vi "Test Program.vi"() -> ()   [LabVIEW 2018]
uses:
  <vilib>/Analysis/Matrix/Datatypes/RealMatrix.ctl
  archive/CAEN_SY527 v3/CAEN_SY527/CAEN globals.vi
  <vilib>/Analysis/Matrix/NI_Matrix.lvlib
panel:
  in  "Mainframe 2":refnum<visa-resource-name>
  in  "Buffer":T1(ring)=enum."None"
  in  "Action":string(combo)
  in  "Read Port":bool
  in  "Predefined Range":T2(ring)
  in  "Combo funcs":bool
  in  "Write Voltage":bool
  in  "Current Limit (mA)":i32
  in  "Write Current Lim":bool
  in  "Read All":bool
  out "Channel+range":string
  in  "Voltage (V)":i32
  out "Codes Output":string
  in  "Connect to Crate":bool
  out "Channel Read as Matrix":T3
  out "Serial Readout":string
  in  "Abort and Clear":bool
  in  "stop":bool
  in  "Range Source":enum16{"Predefined Range", "Selected Range"}(ring)
  in  "Crate":i32=1
  in  "Card":i32
  in  "Channel":i32
  in  "# Channels":i32
  in  "Read Range":bool
  out "Errors":errorcluster
  in  "Mainframe 1":refnum<visa-resource-name>
  # "Select Channel Range to Operate On"
  # "Write Operations"
  # "Read Operations"
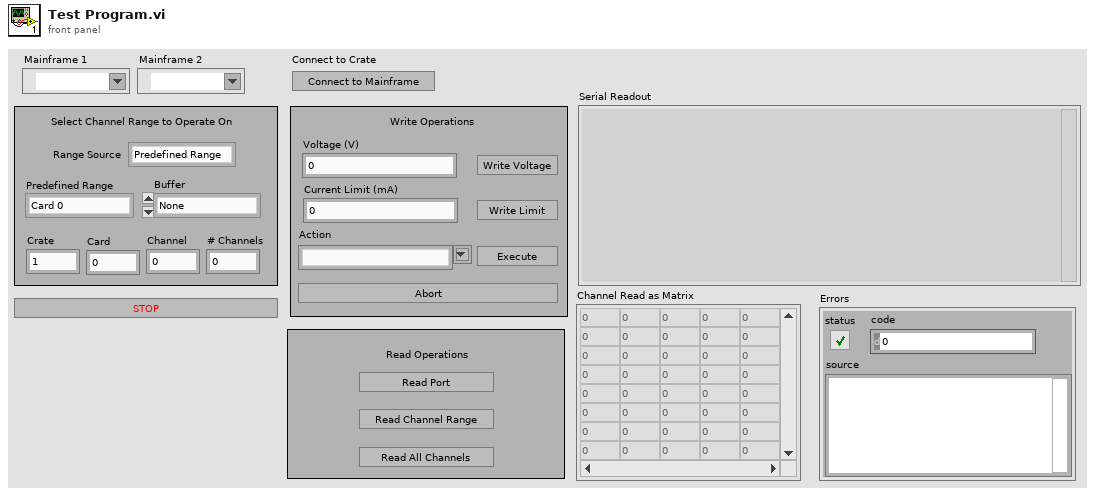
[diagram p1: front panel]
types:
  T1 = enum16{"Monitor", "Demand", "Backup", "All", "None"}
  T2 = enum16{"Card 0", "Card 1", "Card 2", "Card 3", "Card 4", "Card 5", "Card 6", "Card 7", "Card 8", "Card 9", "Card 10", "Card 11", "Card 12", "Card 13", "Card 14", "Card 15"}
  T3 = typedef "NI_Matrix.lvlib/RealMatrix.ctl" = dbl[][]
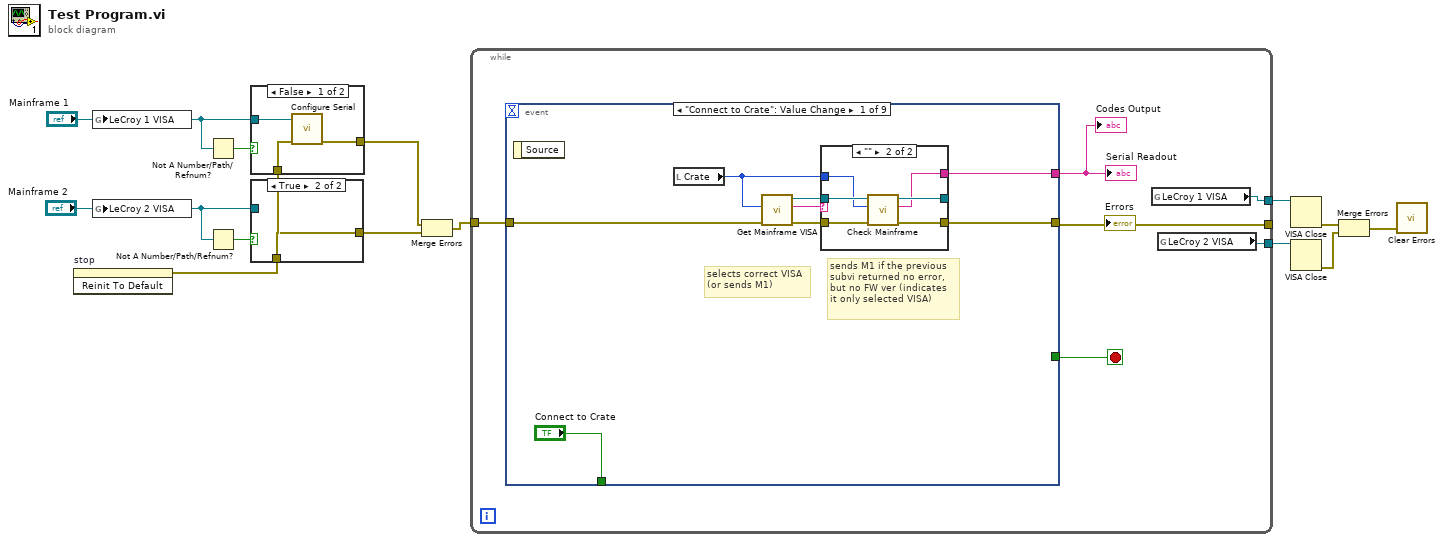
[diagram p0: block diagram]
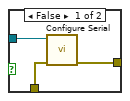
[diagram p2: hidden frame]
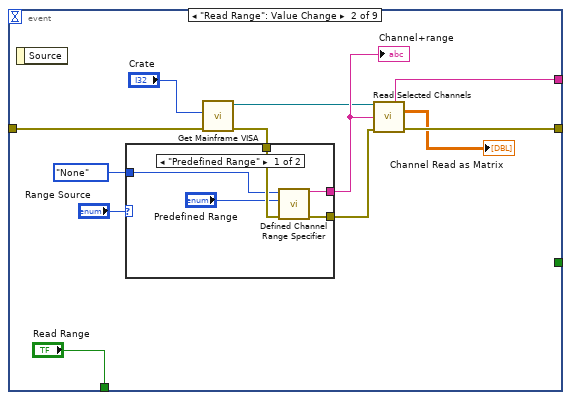
[diagram p5: hidden frame]
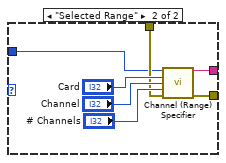
[diagram p6: hidden frame]
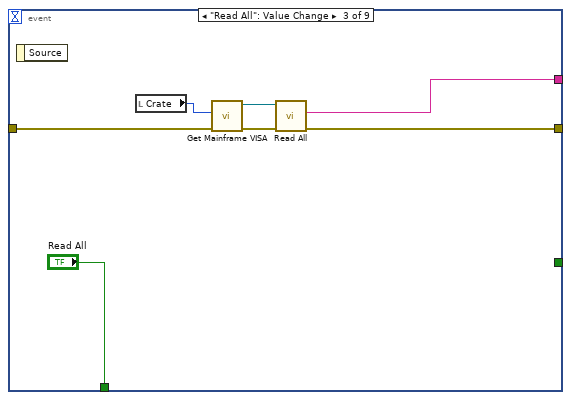
[diagram p7: hidden frame]
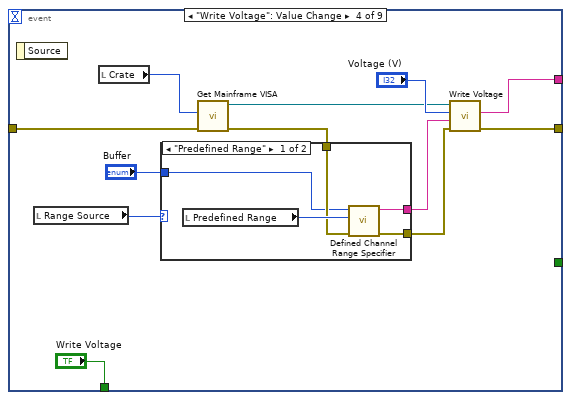
[diagram p8: hidden frame]
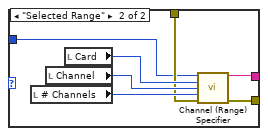
[diagram p9: hidden frame]
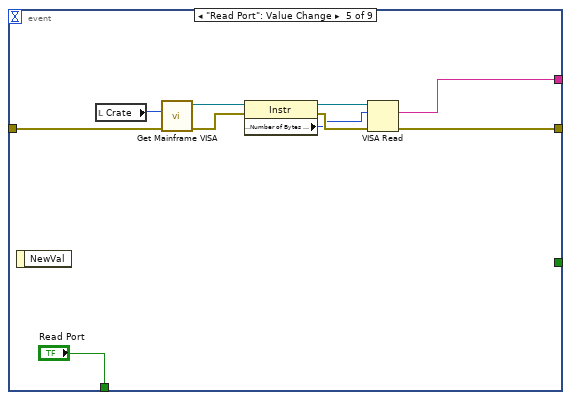
[diagram p10: hidden frame]
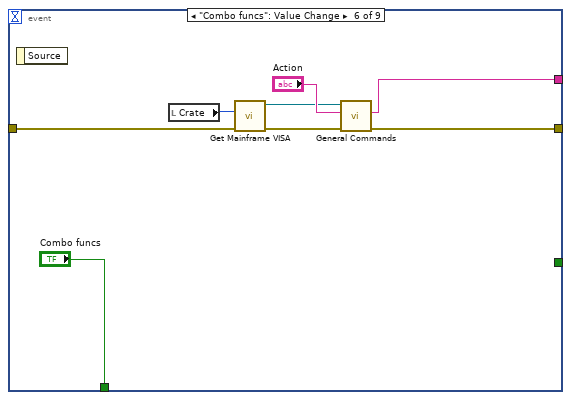
[diagram p11: hidden frame]
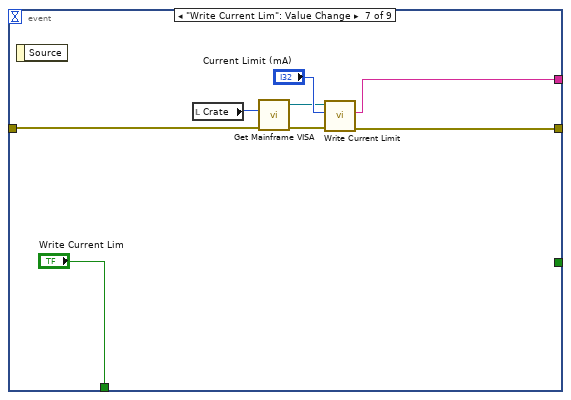
[diagram p12: hidden frame]
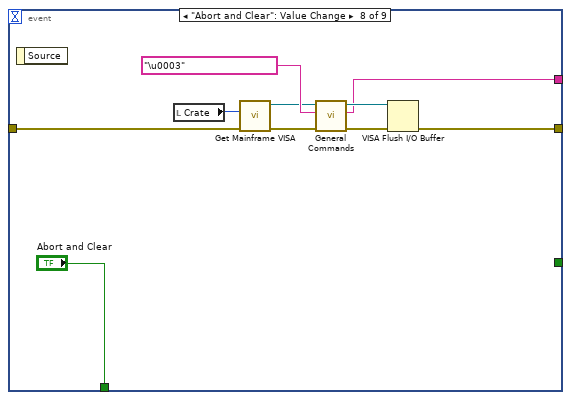
[diagram p13: hidden frame]
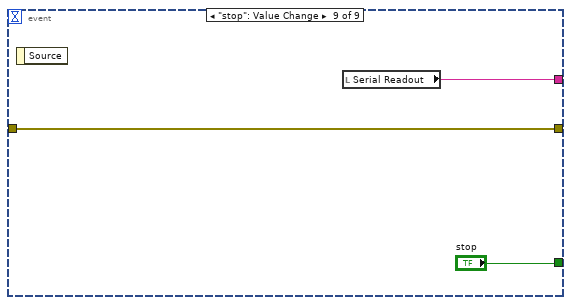
[diagram p14: hidden frame]
diagram:
  n1 = invoke on="stop" class="Bool" method="Reinit To Default"() -> (error out=w11:errorcluster)  [unwired: 3 in, 2 out]
  n2 = global write "CAEN globals.vi" "LeCroy 1 VISA"("Mainframe 1") -> ()
  n3 = global write "CAEN globals.vi" "LeCroy 2 VISA"("Mainframe 2") -> ()
  n4 = Not A Number/Path/Refnum?(number/path/refnum="Mainframe 1") -> (NaN/Path/Refnum?=w7:bool)
  n5 = Not A Number/Path/Refnum?(number/path/refnum="Mainframe 2") -> (NaN/Path/Refnum?=w4:bool)
  n6 = case shown="False" w7 {
    tunnel: "Mainframe 1" -> [w16 _]
    tunnel: w11 -> [w15 w17]
    tunnel: [w14 w17] -> w10
    frame False {
      n7 = call "Configure Serial.vi"("error in"=w15, "Resource Name"=w16) -> ("error out"=w14:errorcluster)  [unwired: 8 in, 1 out]
    }
    frame True {
    }
  }
  n8 = case shown="True" w4 {
    tunnel: "Mainframe 2" -> [w20 _]
    tunnel: w11 -> [w19 w21]
    tunnel: [w18 w21] -> w9
    frame False {
      n9 = call "Configure Serial.vi"("error in"=w19, "Resource Name"=w20) -> ("error out"=w18:errorcluster)  [unwired: 8 in, 1 out]
    }
    frame True {
    }
  }
  n10 = Merge Errors(w10, w9) -> (w8:errorcluster)
  n11 = while {
    tunnel: [w22] -> _
    tunnel: w8 -> [w25]
    tunnel: [w24] -> w3
    tunnel: [w23] -> w2
    stop <- w27 stop-if-true
    n12 = event shown="[0] \"Connect to Crate\": Value Change" {
      selector: _ -> [_ _ _ _ _ _ _ _ _]
      dyn-events: _ -> [_ _ _ _ _ _ _ _ _]
      timeout: _ -> [_ _ _ _ _ _ _ _ _]
      tunnel: [_ _ _ _ _ _ _ _ "stop"] -> w27
      tunnel: w25 -> [w35 w50 w70 w82 w102 w111 w118 w126 w136]
      tunnel: [w31 w55 w75 w86 w105 w117 w125 w134 w136] -> w22
      tunnel: [w30 w54 w74 w83 w104 w116 w123 w130 w135] -> w26
      tunnel: ["Connect to Crate" "Read Range" "Read All" "Write Voltage" "Read Port" "Combo funcs" "Write Current Lim" "Abort and Clear" _] -> _
      event "Connect to Crate": Value Change {
        # "sends M1 if the previous\nsubvi returned no error, \nbut no FW ver (indicates\nit only selected VISA)"
        # "selects correct VISA\n(or sends M1)"
        n13 = event-data() -> ()  [unwired: 1 in, 1 out]
        n14 = local read "Crate"() -> (w28:i32)
        n15 = call "Get Mainframe VISA.vi"("Error In"=w35, "Crate"=w28) -> ("Error Out"=w33:errorcluster, "Version Output"=w29:string, "VISA out"=w32:refnum<visa-resource-name>)  [unwired: 7 in]
        n16 = case shown="\"\"" w29 {
          selector: w29 -> [w36 _]
          tunnel: w33 -> [w37 w44]
          tunnel: w32 -> [w38 w43]
          tunnel: [w37 w42] -> w31
          tunnel: [w38 w41] -> _
          tunnel: [w36 w40] -> w30
          tunnel: w28 -> [_ w39]
          frame Default {
          }
          frame "" {
            n17 = call "Check Mainframe.vi"("error in"=w44, "Mainframe"=w39, "VISA resource name"=w43) -> ("error out"=w42:errorcluster, "Version Output"=w40:string, "VISA resource name out"=w41:refnum<visa-resource-name>)  [unwired: 6 in]
          }
        }
      }
      event "Read Range": Value Change {
        n18 = event-data() -> ()  [unwired: 1 in, 1 out]
        n19 = call "Get Mainframe VISA.vi"("Error In"=w50, "Crate"="Crate") -> ("Error Out"=w47:errorcluster, "VISA out"=w49:refnum<visa-resource-name>)  [unwired: 7 in, 1 out]
        n20 = case shown="\"Predefined Range\"" "Range Source" {
          tunnel: [w60 w65] -> w53
          tunnel: w47 -> [w59 w64]
          tunnel: [w61 w63] -> w46
          tunnel: T1."None" ("Buffer") -> [w57 w62]
          frame "Predefined Range" {
            n21 = call "Defined Channel Range Specifier.vi"("error in"=w59, "Card"="Predefined Range", "Buffer"=w57) -> ("error out"=w61:errorcluster, "Channel Range"=w60:string)  [unwired: 7 in]
          }
          frame "Selected Range" {
            n22 = call "Channel (Range) Specifier.vi"("Buffer"=w62, "Card"="Card", "Channel"="Channel", "Num Channels"="# Channels", "error in"=w64) -> ("Channel (Range)"=w65:string, "error out"=w63:errorcluster)  [unwired: 9 in]
          }
        }
        "Channel+range" <- w53
        n23 = call "Read Selected Channels.vi"("VISA in"=w49, "C##,##DO###"=w53, "error in"=w46) -> ("Final Output"=w54:string, "Channel Array"=→"Channel Read as Matrix":dbl[][], "error out"=w55:errorcluster)  [unwired: 6 in, 4 out]
      }
      event "Read All": Value Change {
        n24 = event-data() -> ()  [unwired: 1 in, 1 out]
        n25 = local read "Crate"() -> (w69:i32)
        n26 = call "Get Mainframe VISA.vi"("Error In"=w70, "Crate"=w69) -> ("Error Out"=w72:errorcluster, "VISA out"=w71:refnum<visa-resource-name>)  [unwired: 7 in, 1 out]
        n27 = call "Read All.vi"("error in"=w72, "VISA Refnum in"=w71) -> ("error out"=w75:errorcluster, "Final Output"=w74:string)  [unwired: 7 in, 1 out]
      }
      event "Write Voltage": Value Change {
        n28 = event-data() -> ()  [unwired: 1 in, 1 out]
        n29 = local read "Range Source"() -> (w84:enum16{"Predefined Range", "Selected Range"})
        n30 = local read "Crate"() -> (w81:i32)
        n31 = call "Get Mainframe VISA.vi"("Error In"=w82, "Crate"=w81) -> ("Error Out"=w78:errorcluster, "VISA out"=w80:refnum<visa-resource-name>)  [unwired: 7 in, 1 out]
        n32 = case shown="\"Predefined Range\"" w84 {
          tunnel: [w90 w99] -> w77
          tunnel: [w92 w95] -> w79
          tunnel: "Buffer" -> [w88 w93]
          tunnel: w78 -> [w89 w94]
          frame "Predefined Range" {
            n33 = local read "Predefined Range"() -> (w91:T2)
            n34 = call "Defined Channel Range Specifier.vi"("error in"=w89, "Card"=w91, "Buffer"=w88) -> ("error out"=w90:errorcluster, "Channel Range"=w92:string)  [unwired: 7 in]
          }
          frame "Selected Range" {
            n35 = local read "# Channels"() -> (w98:i32)
            n36 = local read "Channel"() -> (w97:i32)
            n37 = local read "Card"() -> (w96:i32)
            n38 = call "Channel (Range) Specifier.vi"("Buffer"=w93, "Card"=w96, "Channel"=w97, "Num Channels"=w98, "error in"=w94) -> ("Channel (Range)"=w95:string, "error out"=w99:errorcluster)  [unwired: 9 in]
          }
        }
        n39 = call "Write Voltage.vi"("error in"=w77, "Channel+Range"=w79, "Voltage input"="Voltage (V)", "VISA in"=w80) -> ("error out"=w86:errorcluster, "read buffer"=w83:string)  [unwired: 5 in, 1 out]
      }
      event "Read Port": Value Change {
        n40 = event-data() -> ()  [unwired: 1 in, 1 out]
        n41 = local read "Crate"() -> (w103:i32)
        n42 = call "Get Mainframe VISA.vi"("Error In"=w102, "Crate"=w103) -> ("Error Out"=w101:errorcluster, "VISA out"=w100:refnum<visa-resource-name>)  [unwired: 7 in, 1 out]
        n43 = property class="Instr"(reference=w100, error in=w101) -> (reference out=w108:refnum<visa-resource-name>, error out=w107:errorcluster, "Serial Settings:Number of Bytes at Serial Port"=w106:u32)
        n44 = VISA Read(VISA resource name=w108, byte count=w106, error in (no error)=w107) -> (read buffer=w104:string, error out=w105:errorcluster)  [unwired: 2 out]
      }
      event "Combo funcs": Value Change {
        n45 = event-data() -> ()  [unwired: 1 in, 1 out]
        n46 = local read "Crate"() -> (w113:i32)
        n47 = call "Get Mainframe VISA.vi"("Error In"=w111, "Crate"=w113) -> ("Error Out"=w112:errorcluster, "VISA out"=w110:refnum<visa-resource-name>)  [unwired: 7 in, 1 out]
        n48 = call "General Commands.vi"("error in"=w112, "Action"="Action", "VISA in"=w110) -> ("error out"=w117:errorcluster, "result string"=w116:string)  [unwired: 6 in, 1 out]
      }
      event "Write Current Lim": Value Change {
        n49 = event-data() -> ()  [unwired: 1 in, 1 out]
        n50 = local read "Crate"() -> (w121:i32)
        n51 = call "Get Mainframe VISA.vi"("Error In"=w118, "Crate"=w121) -> ("Error Out"=w120:errorcluster, "VISA out"=w119:refnum<visa-resource-name>)  [unwired: 7 in, 1 out]
        n52 = call "Write Current Limit.vi"("error in"=w120, "Current Limit (mA)"="Current Limit (mA)", "VISA in"=w119) -> ("error out"=w125:errorcluster, "Output"=w123:string)  [unwired: 6 in, 1 out]
      }
      event "Abort and Clear": Value Change {
        n53 = event-data() -> ()  [unwired: 1 in, 1 out]
        n54 = local read "Crate"() -> (w129:i32)
        n55 = call "Get Mainframe VISA.vi"("Error In"=w126, "Crate"=w129) -> ("Error Out"=w128:errorcluster, "VISA out"=w127:refnum<visa-resource-name>)  [unwired: 7 in, 1 out]
        n56 = call "General Commands.vi"("error in"=w128, "Action"="\u0003", "VISA in"=w127) -> ("error out"=w134:errorcluster, "result string"=w130:string, "VISA out"=w133:refnum<visa-resource-name>)  [unwired: 6 in]
        n57 = VISA Flush I/O Buffer(VISA resource name=w133) -> ()  [unwired: 2 in, 2 out]
      }
      event "stop": Value Change {
        n58 = event-data() -> ()  [unwired: 1 in, 1 out]
        n59 = local read "Serial Readout"() -> (w135:string)
      }
    }
    "Serial Readout" <- w26
    "Codes Output" <- w26
    "Errors" <- w22
    n60 = global read "CAEN globals.vi" "LeCroy 1 VISA"() -> (w24:refnum<visa-resource-name>)
    n61 = global read "CAEN globals.vi" "LeCroy 2 VISA"() -> (w23:refnum<visa-resource-name>)
  }
  n62 = VISA Close(VISA resource name=w3) -> (error out=w13:errorcluster)  [unwired: 1 in]
  n63 = VISA Close(VISA resource name=w2) -> (error out=w12:errorcluster)  [unwired: 1 in]
  n64 = Merge Errors(w13, w12) -> (w1:errorcluster)
  n65 = call <vilib>:"Clear Errors.vi"("error in (no error)"=w1) -> ()  [unwired: 5 in, 2 out]
